vi "数组索引.vi"() -> ()   [LabVIEW 2020]
doc: "本VI是为《我和LabVIEW》一书编写的示例。\n关于本书的介绍请参考网页：\nhttp://ruanqizhen.spaces.live.com/blog/cns!5852D4F797C53FB6!4310.entry"
panel:
  out "元素[2][1]":string
  out "第一列":string[](array[string])
  out "第一行":string[](array[string])
  out "元素 3":string
  out "元素 2":string
  out "元素 1":string
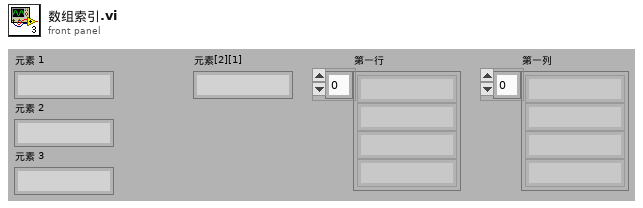
[diagram p1: front panel]
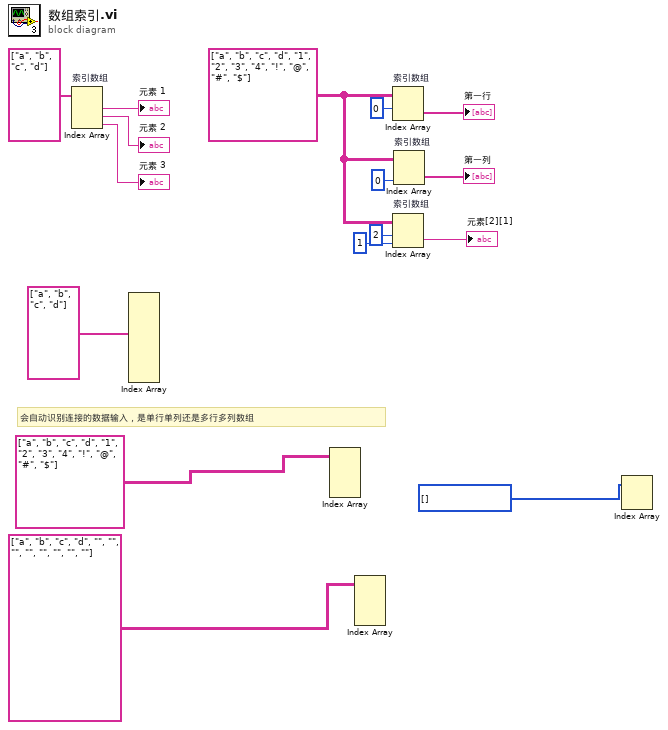
[diagram p0: block diagram]
diagram:
  w7 = string[][] [["a", "b", "c", "d"], ["1", "2", "3", "4"], ["!", "@", "#", "$"]] ("数组")
  # "会自动识别连接的数据输入，是单行单列还是多行多列数组"
  n1 = Index Array "索引数组"(array=string[] ["a", "b", "c", "d"] ("数组")) -> (element #1=→"元素 1":string, element #2=→"元素 2":string, element #3=→"元素 3":string)  [unwired: 3 in]
  n2 = Index Array(array=string[] ["a", "b", "c", "d"] ("数组")) -> ()  [unwired: 9 in, 9 out]
  n3 = Index Array(array=string[][] [["a", "b", "c", "d"], ["1", "2", "3", "4"], ["!", "@", "#", "$"]] ("数组")) -> ()  [unwired: 4 in, 2 out]
  n4 = Index Array(array=string[][] [["a", "b", "c", "d"], ["", "", "", ""], ["", "", "", ""]] ("数组")) -> ()  [unwired: 4 in, 2 out]
  n5 = Index Array "索引数组"(array=w7, index (row)=0 ("索引 (行)")) -> (element=→"第一行":string[])  [unwired: 1 in]
  n6 = Index Array "索引数组"(array=w7, index (row)=2 ("禁用的索引 (行)"), index (col)=1 ("禁用的索引 (列)")) -> (element=→"元素[2][1]":string)
  n7 = Index Array "索引数组"(array=w7, index (col)=0 ("禁用的索引 (列)")) -> (element=→"第一列":string[])  [unwired: 1 in]
  n8 = Index Array(array=i32[] []) -> ()  [unwired: 2 in, 2 out]
